vi "Add Event.vi"(0 "CurrentEvents In":T1[](array[typedef]), 2 "Event":T1) -> (4 "CurrentEvents out":T1[](array[typedef]))   [LabVIEW 2019, in "Logger.lvclass"]
uses:
  Logger.lvclass
  EventData.ctl
  TypeDef/AlarmType.ctl
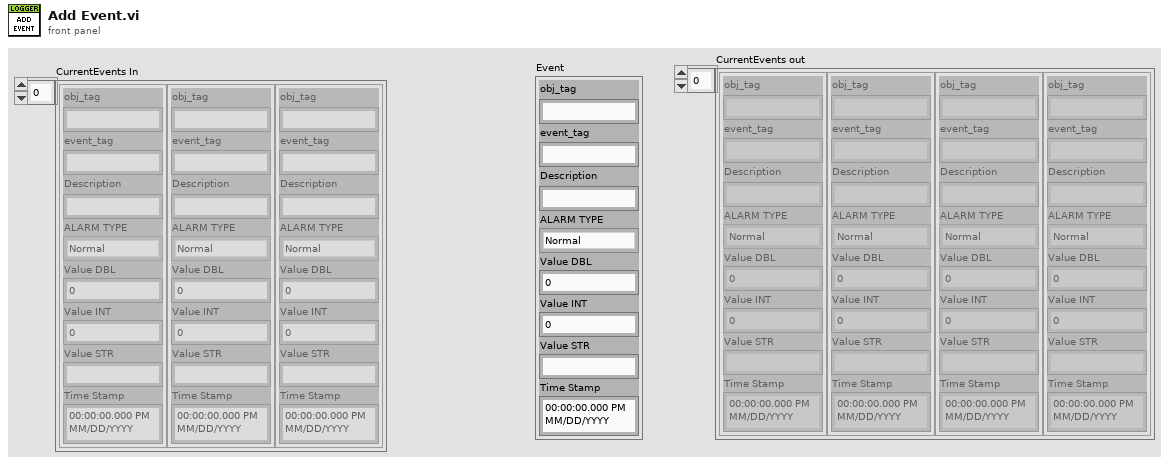
[diagram p1: front panel]
types:
  T1 = typedef "EventData.ctl" = cluster{"obj_tag":string, "event_tag":string, "Description":string, "ALARM TYPE":T2, "Value DBL":dbl, "Value INT":i32, "Value STR":string, "Time Stamp":timestamp}
  T2 = typedef "AlarmType.ctl" = enum16{"Normal", "Warning", "Alarm"}
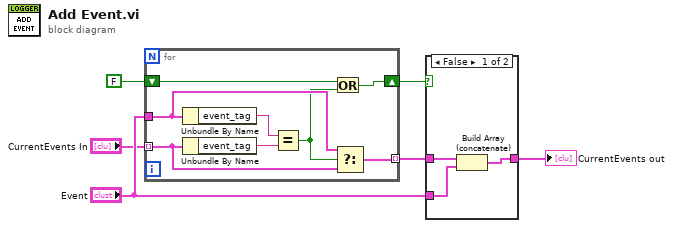
[diagram p0: block diagram]
diagram:
  n1 = for {
    tunnel: "CurrentEvents In" -> [w11] mode=indexing
    tunnel: "Event" -> [w12]
    tunnel: [w10] -> w3 mode=indexing
    shift-right: [w8] -> w5
    shift-left: FALSE -> [w7]
    n2 = Unbundle By Name(w12) -> ("event_tag"=w13:string)
    n3 = Unbundle By Name(w11) -> ("event_tag"=w14:string)
    n4 = Equal?(x=w13, y=w14) -> (x = y?=w9:bool)
    n5 = Or(x=w7, y=w9) -> (x .or. y?=w8:bool)
    n6 = Select(t=w12, s=w9, f=w11) -> (s? t:f=w10:T1)
  }
  n7 = case shown="False" w5 {
    tunnel: w3 -> [w17 w18]
    tunnel: [w16 w18] -> w4
    tunnel: "Event" -> [w15 _]
    frame False {
      n8 = Build Array (concatenate)(w17, w15) -> (w16:T1[])
    }
    frame True {
    }
  }
  "CurrentEvents out" <- w4
